vi "Configure Trigger Slope1.vi"(8 "error in (no error)":errorcluster, 10 "Trigger Edge (1: Negative)":i32(ring)=1 items=["Positive", "Negative"], 11 "VISA resource name":refnum<visa-resource-name>) -> (0 "error out":errorcluster, 3 "VISA resource name out":refnum<visa-resource-name>)   [LabVIEW 2015, in "Agilent 3446X Series1.lvlib"]
doc: "Configures whether the instrument uses the rising edge (POS) or the falling edge (NEG) of the trigger signal on the rearpanel Ext Trig BNC connector."
uses:
  Agilent 3446X Series1.lvlib
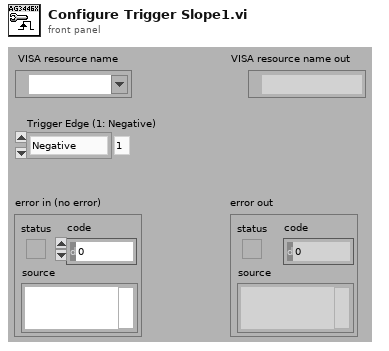
[diagram p1: front panel]
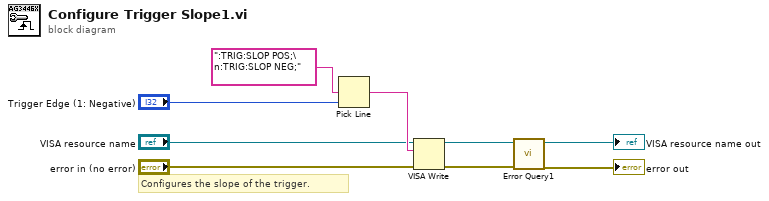
[diagram p0: block diagram]
diagram:
  # "Configures the slope of the trigger."
  n1 = Pick Line(multi-line string=":TRIG:SLOP POS;\n:TRIG:SLOP NEG;", line index="Trigger Edge (1: Negative)") -> (output string=w7:string)  [unwired: 1 out]
  n2 = VISA Write(VISA resource name="VISA resource name", write buffer=w7, error in (no error)="error in (no error)") -> (VISA resource name out=w4:refnum<visa-resource-name>, error out=w3:errorcluster)  [unwired: 1 out]
  n3 = call "Error Query1.vi"("error in (no error)"=w3, "VISA resource name"=w4) -> ("error out"=→"error out":errorcluster, "VISA resource name out"=→"VISA resource name out":refnum<visa-resource-name>)  [unwired: 8 out]
